vi "GEOM_GUI_tcp_server.vi"(4 "resp queue":refnum<queue>, 6 "from sock queue":refnum<queue>, 10 "port":u16) -> ()   [LabVIEW 2016]
doc: "Handles the asynchronous messages coming from the TCS, as well as the responses for commands which requieres a long time for completion"
panel:
  out "listener ID out":refnum<k5>
  out "stop":bool
  out "sock ID":refnum<k5>
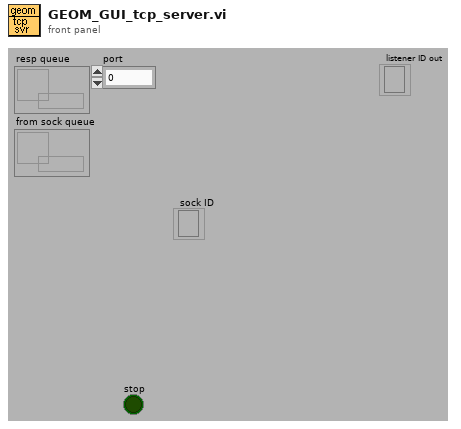
[diagram p1: front panel]
types:
  T1 = enum16{"Standard", "Buffered", "CRLF", "Immediate"}
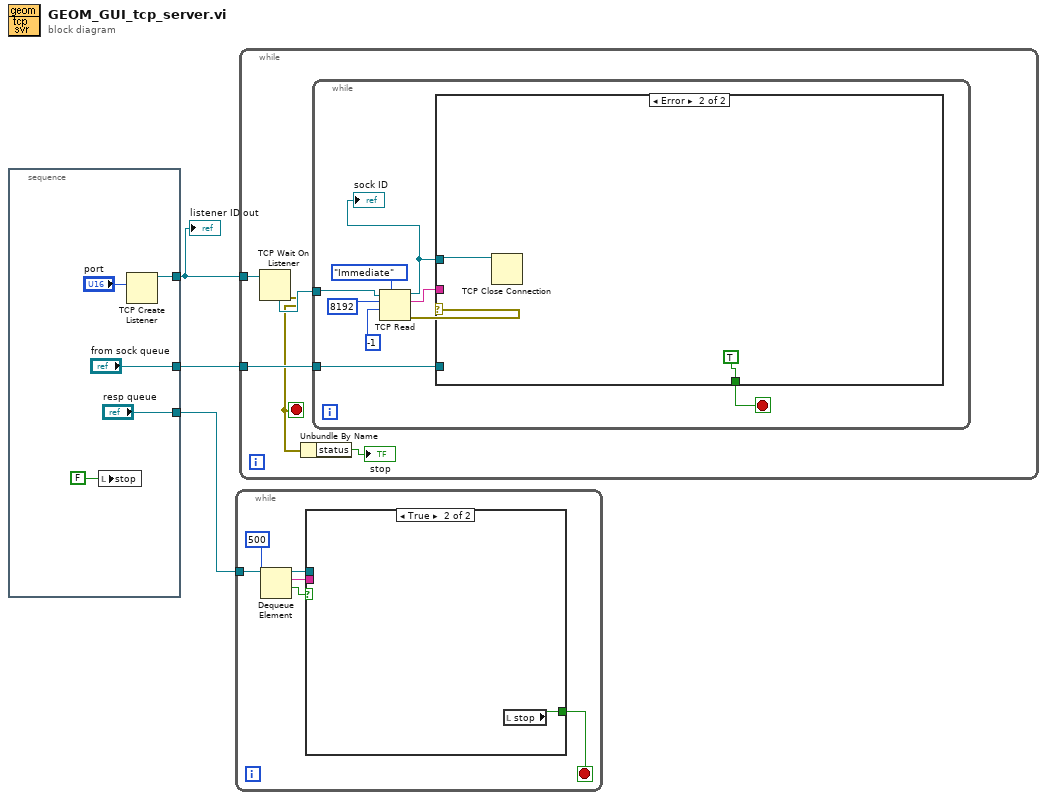
[diagram p0: block diagram]
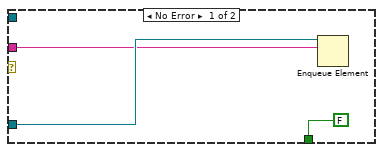
[diagram p2: hidden frame]
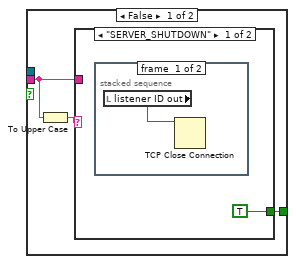
[diagram p3: hidden frame]
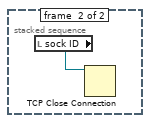
[diagram p4: hidden frame]
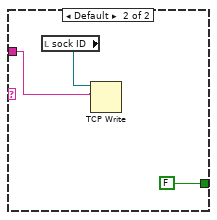
[diagram p5: hidden frame]
diagram:
  n1 = stacked-sequence {
    tunnel: ["resp queue"] -> w3
    tunnel: ["from sock queue"] -> w2
    tunnel: [w4] -> w1
    frame #0 {
      n2 = local write "stop"(FALSE ("stop")) -> ()
      n3 = TCP Create Listener(10:"port") -> (3:w4:refnum<k5>)  [unwired: 1 in, 5 out]
    }
  }
  "listener ID out" <- w1
  n4 = while {
    tunnel: w3 -> [w14]
    stop <- w13 stop-if-true
    n5 = Dequeue Element(queue=w14, timeout in ms (-1)=500) -> (queue out=w12:refnum<queue>, element=w10:string, timed out?=w9:bool)  [unwired: 1 in, 1 out]
    n6 = case shown="True" w9 {
      tunnel: w10 -> [w16 _]
      tunnel: [w17 w24] -> w13
      tunnel: w12 -> [_ _]
      frame False {
        n7 = To Upper Case(1:w16) -> (0:w15:string)
        n8 = case shown="\"SERVER_SHUTDOWN\"" w15 {
          tunnel: w16 -> [_ w23]
          tunnel: [TRUE FALSE] -> w17
          frame "SERVER_SHUTDOWN" {
            n9 = stacked-sequence {
              frame #0 {
                n10 = local read "listener ID out"() -> (w19:refnum<k5>)
                n11 = TCP Close Connection(connection ID=w19) -> ()  [unwired: 1 in, 3 out]
              }
              frame #1 {
                n12 = local read "sock ID"() -> (w20:refnum<k5>)
                n13 = TCP Close Connection(connection ID=w20) -> ()  [unwired: 1 in, 3 out]
              }
            }
          }
          frame Default {
            n14 = local read "sock ID"() -> (w21:refnum<k5>)
            n15 = TCP Write(connection ID=w21, data in=w23) -> ()  [unwired: 1 in, 4 out]
          }
        }
      }
      frame True {
        n16 = local read "stop"() -> (w24:bool)
      }
    }
  }
  n17 = while {
    tunnel: w2 -> [w29]
    tunnel: w1 -> [w28]
    stop <- w26 stop-if-true
    n18 = TCP Wait On Listener(11:w28) -> (0:w26:errorcluster, 4:w27:refnum<k5>)  [unwired: 1 in, 5 out]
    n19 = Unbundle By Name(w26) -> ("status"=→"stop":bool)
    n20 = while {
      tunnel: w27 -> [w32]
      tunnel: w29 -> [w33]
      stop <- w30 stop-if-true
      n21 = TCP Read(connection ID=w32, bytes to read=8192, 7:T1."Immediate" ("mode (standard)"), 9:-1 ("timeout ms (25000)")) -> (connection ID out=w31:refnum<k5>, data out=w34:string, error out=w36:errorcluster)  [unwired: 1 in]
      "sock ID" <- w31
      n22 = case shown="Error" w36 {
        tunnel: w34 -> [w39 _]
        tunnel: [FALSE TRUE] -> w30
        tunnel: w31 -> [_ w42]
        tunnel: w33 -> [w40 _]
        frame No Error {
          n23 = Enqueue Element(queue=w40, element=w39) -> ()  [unwired: 1 in, 4 out]
        }
        frame Error {
          n24 = TCP Close Connection(connection ID=w42) -> ()  [unwired: 1 in, 3 out]
        }
      }
    }
  }
